vi "Set Cell View.vi"(7 "Cell View":refnum<class "Cell View.lvclass">, 8 "error in":errorcluster, 9 "Column":i32, 10 "Row":i32, 11 "SourceGrid in":refnum<class "SourceGrid.lvclass">) -> (0 "error out":errorcluster, 3 "SourceGrid out":refnum<class "SourceGrid.lvclass">)   [LabVIEW 2024, in "SourceGrid.lvlib" / "SourceGrid.lvclass"]
uses:
  SourceGrid.lvclass
  Views/Cell View/Cell View.lvclass
  SourceGrid.lvclass/SourceGrid.ctl
  Views/Cell View/Cell View.lvclass/Cell View.ctl
  D:/git/Sourcegrid-LabVIEW/dll/SourceGrid.dll
  dll/SourceGrid.dll
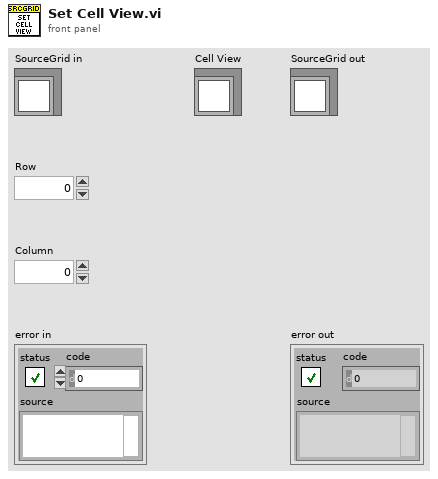
[diagram p1: front panel]
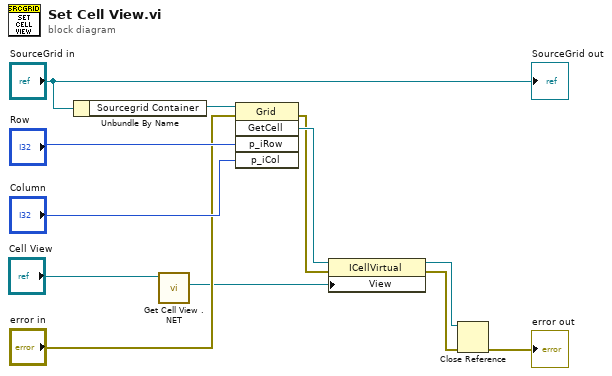
[diagram p0: block diagram]
diagram:
  n1 = Unbundle By Name("SourceGrid in") -> ("Sourcegrid Container"=w11:refnum<k24>)
  n2 = call "Get Cell View .NET.vi"("Cell View in"="Cell View") -> ("Cell View .NET"=w4:refnum<k24>)  [unwired: 9 in, 1 out]
  n3 = invoke class="Grid" method="GetCell"(reference=w11, error in="error in", "p_iRow"="Row", "p_iCol"="Column") -> (error out=w3:errorcluster, "GetCell"=w5:refnum<k24>)  [unwired: 1 in, 3 out]
  n4 = property class="ICellVirtual"(reference=w5, error in=w3, "View"=w4) -> (reference out=w1:refnum<k24>, error out=w2:errorcluster)
  n5 = Close Reference(reference=w1, error in (no error)=w2) -> (error out=→"error out":errorcluster)
  "SourceGrid out" <- "SourceGrid in"
